vi "DB UI - MasterData SAPMaterial (Long) Description.vi"(6 "FP is Modal":bool, 7 "DB Connection":T3={"Open"=TRUE, "Close"=TRUE}, 8 "error in (no error)":errorcluster, 9 "[LanguageId]":string, 10 "[MaterialNo]":string, 11 "connection reference 2":T1) -> (0 "SUMMARY":errorcluster, 2 "[Description] (Long)":string caption="Long Text", 3 "connection reference":T1)   [LabVIEW 2013]
uses:
  <vilib>/addons/database/Connection.llb/Conn ObjectReference.ctl
  Controls/DB - OpenClose.ctl
  <vilib>/Utility/miscctls.llb/LVPointTypeDef.ctl
  Controls/Global SRTRS.vi
  <vilib>/addons/database/Connection.llb/DB Tools Open Connec (String).vi
  <vilib>/addons/database/NI_Database_API.lvlib
panel:
  in  "Tab Control":enum32{"Debug"}(tab)
  out "Connection Information":T2={"Connection "="SQL Server 32bit HPEnvy", "Username"="admin", "Password"="admin123"}
  in  "SRTRS.MasterData.SAPMaterial":string="SRTRS.MasterData.SAPMaterial"
  out "SQL Statement":string
  out "Close 2":errorcluster
  out "FP":errorcluster
  in  "Close":bool caption="Setup Save"
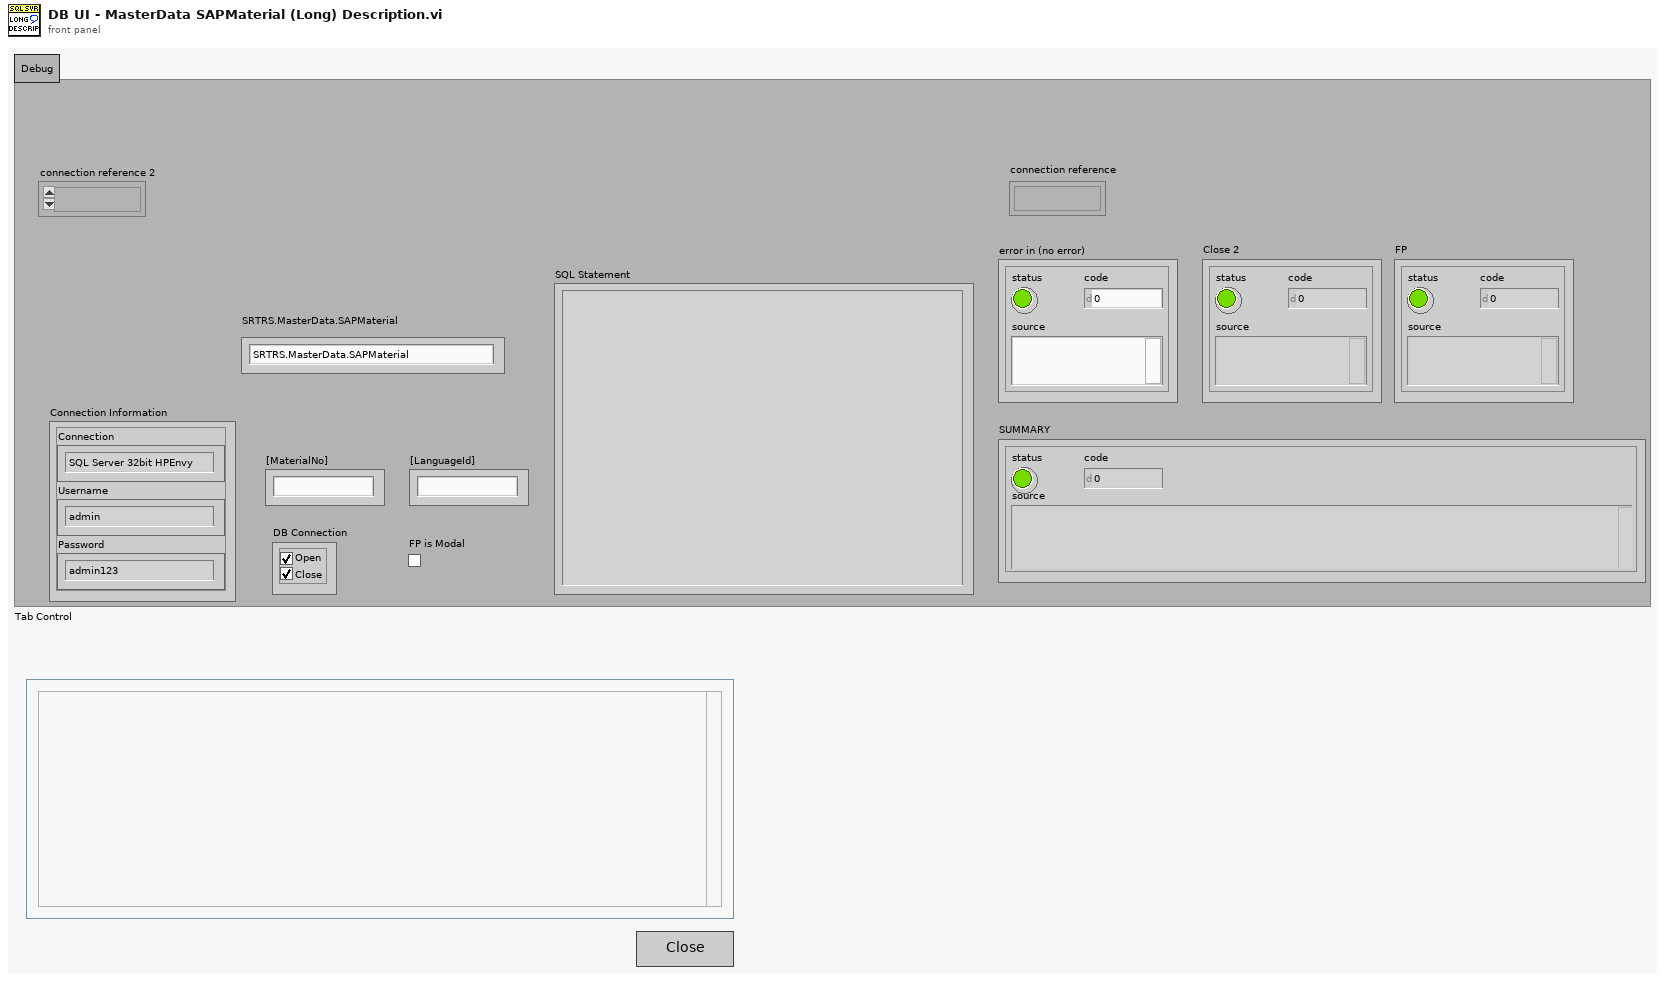
[diagram p1: front panel]
types:
  T1 = typedef "NI_Database_API.lvlib/Conn ObjectReference.ctl" = refnum<k1>
  T2 = cluster{"Connection ":string, "Username":string, "Password":string}
  T3 = typedef "DB - OpenClose.ctl" = cluster{"Open":bool, "Close":bool}
  T4 = typedef "LVPointTypeDef.ctl" = cluster{"Horizontal":i16, "Vertical":i16}
  T5 = typedef "Enum - InteractiveMode-SubVIMode.ctl" = enum16{"Interactive", "subVI Mode"}
  T6 = typedef "DB - DB.Schema.Table.ctl" = cluster{"DB":string, "Schema":string, "Table":string}
  T7 = typedef "Connection Information Cluster.ctl" = cluster{"Connection ":string, "Username":string, "Password":string}
  T8 = typedef "DB - Logon Extra Info.ctl" = cluster{"Plant Name":string, "UserName":string, "Hostname [ClientName]":string, "IsUnicode":bool}
  T9 = enum32{"Invalid", "Default", "Floating", "Floating/Auto-Hide", "Modal"}
  T10 = enum32{"Invalid", "Standard", "Closed", "Hidden", "Minimized", "Maximized"}
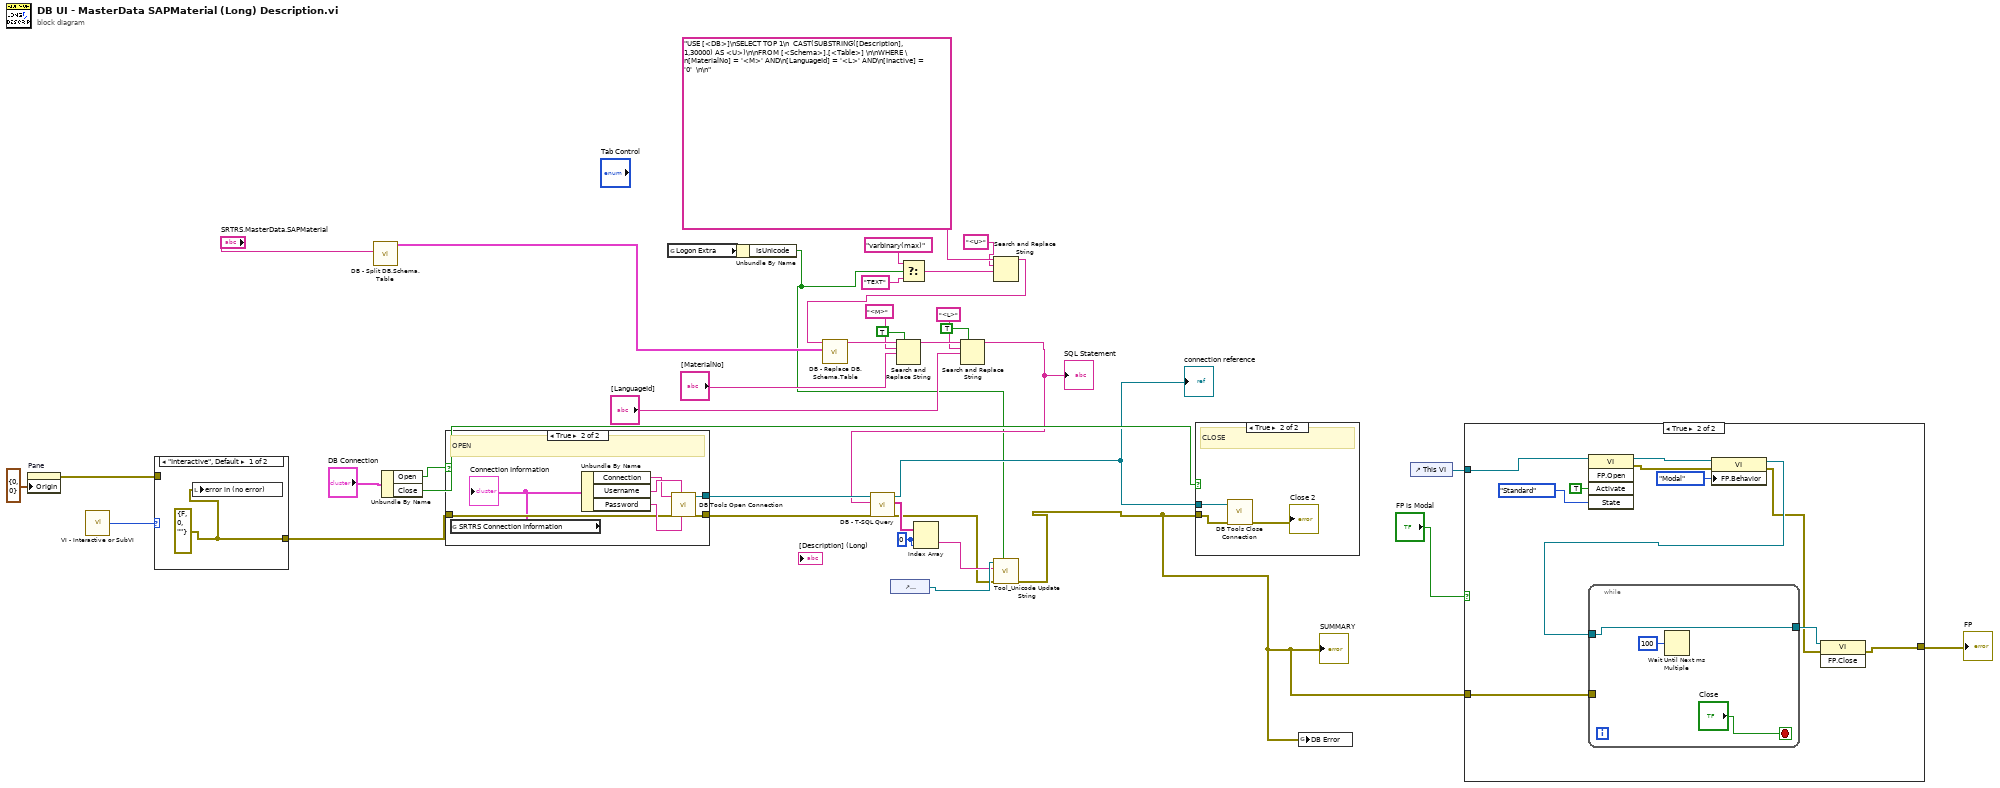
[diagram p0: block diagram]
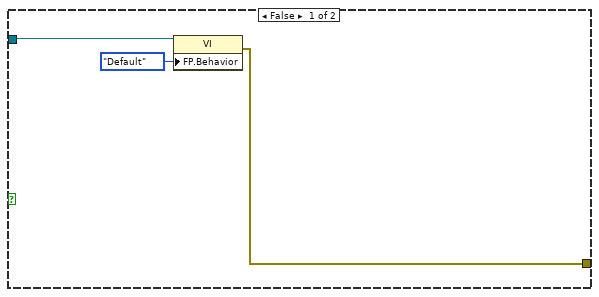
[diagram p2: hidden frame]
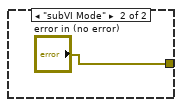
[diagram p4: hidden frame]
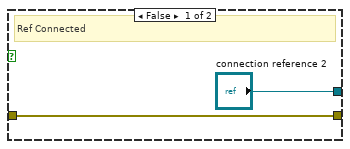
[diagram p5: hidden frame]
diagram:
  w23 = 0 ("index (row)")
  n1 = property on="Pane" class="Pane"("Origin"=T4 {"Horizontal"=0, "Vertical"=0}) -> (error out=w27:errorcluster)  [unwired: 2 in, 1 out]
  n2 = call "VI - Interactive or SubVI.vi"() -> ("Mode"=w36:T5)  [unwired: 5 in]
  n3 = case shown="\"Interactive\", Default" w36 {
    tunnel: [w39 "error in (no error)"] -> w35
    tunnel: w27 -> [_ _]
    frame "Interactive", Default {
      w39 = errorcluster {"status"=FALSE, "code"=0, "source"=""} ("error in (no error)")
      n4 = local write "error in (no error)"(w39) -> ()
    }
    frame "subVI Mode" {
    }
  }
  n5 = call "DB - Split DB.Schema.Table.vi"("DB.Schema.Table"="SRTRS.MasterData.SAPMaterial") -> ("DB.Schema.Table"=w32:T6)  [unwired: 10 in]
  n6 = Unbundle By Name("DB Connection") -> ("Open"=w37:bool, "Close"=w34:bool)
  n7 = case shown="True" w37 {
    tunnel: ["connection reference 2" w46] -> w26
    tunnel: w35 -> [w41 w45]
    tunnel: [w41 w44] -> w25
    frame False {
      # "Ref Connected"
    }
    frame True {
      # "OPEN"
      n8 = global read "Global SRTRS.vi" "SRTRS Connection Information"() -> (w43:T7)
      "Connection Information" <- w43
      n9 = Unbundle By Name(w43) -> ("Connection"=w48:string, "Username"=w49:string, "Password"=w47:string)
      n10 = call-poly <vilib>:"DB Tools Open Connection.vi"("password"=w47, "userID"=w49, "error in (no error)"=w45, "connection information"=w48) -> ("error out"=w44:errorcluster, "connection reference"=w46:T1)  [unwired: 4 in]
    }
  }
  n11 = global read "Global SRTRS.vi" "Logon Extra"() -> (w2:T8)
  n12 = Unbundle By Name(w2) -> ("IsUnicode"=w1:bool)
  n13 = control-ref of="[Description] (Long)"() -> (w6:refnum<vi>)
  n14 = Select(t="varbinary(max)", s=w1, f="TEXT") -> (s? t:f=w10:string)
  n15 = Search and Replace String(input string="USE [<DB>]\nSELECT TOP 1\n  CAST(SUBSTRING([Description], 1,30000) AS <U>)\n\nFROM [<Schema>].[<Table>] \n\nWHERE \n[MaterialNo] = '<M>' AND\n[LanguageId] = '<L>' AND\n[Inactive] = '0'  \n\n", search string="<U>", replace string=w10) -> (result string=w8:string)  [unwired: 5 in, 3 out]
  n16 = call "DB - Replace DB.Schema.Table.vi"("DB.Schema.Table"=w32, "string in"=w8) -> ("string out"=w31:string)  [unwired: 8 in, 1 out]
  n17 = Search and Replace String(replace all?=TRUE ("replace all? (F)"), input string=w31, search string="<M>", replace string="[MaterialNo]") -> (result string=w21:string)  [unwired: 4 in, 3 out]
  n18 = Search and Replace String(replace all?=TRUE ("replace all? (F)"), input string=w21, search string="<L>", replace string="[LanguageId]") -> (result string=w20:string)  [unwired: 4 in, 3 out]
  "SQL Statement" <- w20
  n19 = call "DB - T-SQL Query.vi"("error in (no error)"=w25, "T-SQL"=w20, "connection reference"=w26) -> ("error out"=w4:errorcluster, "2D data"=w24:string[][], "connection reference"=w16:T1)  [unwired: 6 in]
  "connection reference" <- w16
  n20 = Index Array(array=w24, index (row)=w23, index (col)=w23) -> (element=w5:string)
  n21 = call "Tool_Unicode Update String.vi"("Interpret as Unicode (T)"=w1, "error in (no error)"=w4, "String Value"=w5, "String Control Reference"=w6) -> ("error out"=w3:errorcluster)  [unwired: 4 in, 1 out]
  "SUMMARY" <- w3
  n22 = case shown="True" w34 {
    tunnel: w16 -> [_ w52]
    tunnel: w3 -> [_ w51]
    frame False {
      # "Ref Connected"
    }
    frame True {
      # "CLOSE"
      n23 = call <vilib>:"DB Tools Close Connection.vi"("error in (no error)"=w51, "connection reference"=w52) -> ("error out"=→"Close 2":errorcluster)  [unwired: 5 in]
    }
  }
  n24 = global write "Global SRTRS.vi" "DB Error"(w3) -> ()
  n25 = control-ref of="This VI"() -> (w15:refnum<vi>)
  n26 = case shown="True" "FP is Modal" {
    tunnel: w3 -> [_ w66]
    tunnel: w15 -> [w54 w65]
    tunnel: [w53 w61] -> w14
    frame False {
      n27 = property class="VI"(reference=w54, "FP.Behavior"=T9."Default" ("Front Panel Window:Behavior")) -> (error out=w53:errorcluster)  [unwired: 1 in, 1 out]
    }
    frame True {
      n28 = invoke class="VI" method="FP.Open"(reference=w65, "Activate"=TRUE ("Activate?"), "State"=T10."Standard") -> (reference out=w60:refnum<vi>, error out=w59:errorcluster)  [unwired: 2 in, 3 out]
      n29 = property class="VI"(reference=w60, error in=w59, "FP.Behavior"=T9."Modal" ("Front Panel Window:Behavior")) -> (reference out=w58:refnum<vi>, error out=w56:errorcluster)
      n30 = while {
        tunnel: w66 -> [_]
        tunnel: w58 -> [w67]
        tunnel: [w67] -> w62
        stop <- "Close" stop-if-true
        n31 = Wait Until Next ms Multiple(millisecond multiple=u32 100) -> ()  [unwired: 1 out]
      }
      n32 = invoke class="VI" method="FP.Close"(reference=w62, error in=w56) -> (error out=w61:errorcluster)  [unwired: 1 in, 2 out]
    }
  }
  "FP" <- w14
